vi "CheckForCommand.vi"(7 "Move to Front? (T)":bool=TRUE, 8 "error in":errorcluster, 10 "Search Command":string="EVM Queue", 11 "Queue in":T1) -> (0 "error out":errorcluster, 2 "Command Found?":bool, 3 "Queue (dup)":T1)   [LabVIEW 2010]
doc: "This VI finds the specific command in the queue and move it to the front of the queue"
uses:
  <userlib>/Common/Queue with Cluster/TYP_Queue with Cluster Reference.ctl
  <userlib>/Common/Queue with Cluster/Enqueue - Multiple Clusters.vi
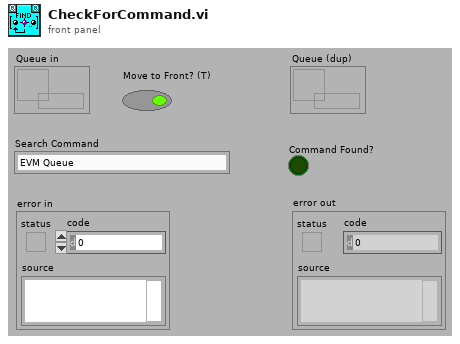
[diagram p1: front panel]
types:
  T1 = typedef "TYP_Queue with Cluster Reference.ctl" = refnum<queue>
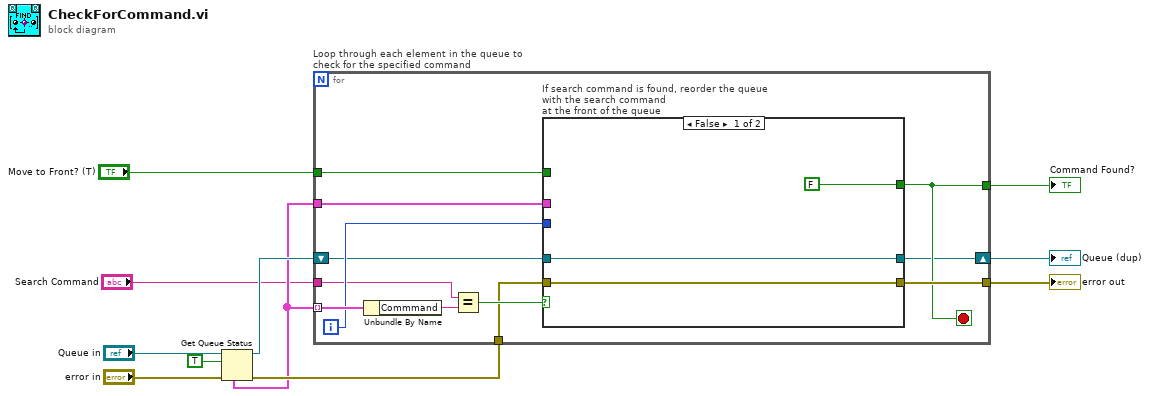
[diagram p0: block diagram]
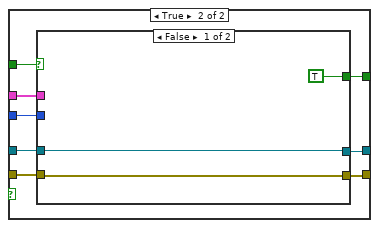
[diagram p2: hidden frame]
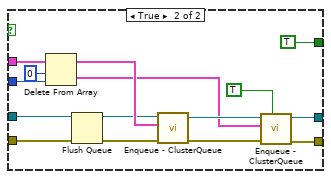
[diagram p3: hidden frame]
diagram:
  n1 = Get Queue Status(queue="Queue in", return elements? (F)=TRUE, error in (no error)="error in") -> (queue out=w10:T1, error out=w11:errorcluster, elements=w9:cluster{"Commmand":string, "Data":variant}[])  [unwired: 5 out]
  n2 = for "Loop through each element in the queue to check for the specified command" {
    tunnel: w9 -> [w23] mode=indexing
    tunnel: w9 -> [w20]
    tunnel: w11 -> [w17]
    tunnel: [w16] -> w4
    tunnel: "Search Command" -> [w15]
    tunnel: [w14] -> w3
    tunnel: "Move to Front? (T)" -> [w13]
    shift-right: [w12] -> w1
    shift-left: w10 -> [w18]
    i -> [w19]
    stop <- w14 stop-if-true
    n3 = Unbundle By Name(w23) -> ("Commmand"=w22:string)
    n4 = Equal?(x=w15, y=w22) -> (x = y?=w21:bool)
    n5 = case "If search command is found, reorder the queue with the search command\nat the front of the queue" shown="False" w21 {
      tunnel: w20 -> [_ w34]
      tunnel: w19 -> [_ w33]
      tunnel: w18 -> [w26 w29]
      tunnel: w17 -> [w25 w28]
      tunnel: [w26 w32] -> w12
      tunnel: [w25 w31] -> w16
      tunnel: [FALSE w30] -> w14
      tunnel: w13 -> [_ w27]
      frame False {
      }
      frame True {
        n6 = case shown="False" w27 {
          tunnel: w34 -> [_ w52]
          tunnel: w33 -> [_ w51]
          tunnel: [w36 w48] -> w32
          tunnel: [w35 w47] -> w31
          tunnel: [TRUE TRUE] -> w30
          tunnel: w29 -> [w36 w41]
          tunnel: w28 -> [w35 w40]
          frame False {
          }
          frame True {
            n7 = Delete From Array(array=w52, length=0, index=w51) -> (deleted portion=w44:cluster{"Commmand":string, "Data":variant}[], array with subset deleted=w49:cluster{"Commmand":string, "Data":variant}[])
            n8 = Flush Queue(queue=w41, error in (no error)=w40) -> (queue out=w39:T1, error out=w38:errorcluster)  [unwired: 1 out]
            n9 = call-poly <userlib>:"Enqueue - ClusterQueue.vi"("error in"=w38, "Array of Clusters"=w49, "Queue with Cluster Reference"=w39) -> ("error out"=w45:errorcluster, "Queue (dup)"=w46:T1)  [unwired: 7 in]
            n10 = call-poly <userlib>:"Enqueue - ClusterQueue.vi"("At Front?"=TRUE, "error in"=w45, "Array of Clusters"=w44, "Queue with Cluster Reference"=w46) -> ("error out"=w47:errorcluster, "Queue (dup)"=w48:T1)  [unwired: 6 in]
          }
        }
      }
    }
  }
  "error out" <- w4
  "Queue (dup)" <- w1
  "Command Found?" <- w3
